vi "GT Get Pos.vi"(8 "error in (no error)":errorcluster caption="错误输入（无错误）", 9 "pPos":i32, 10 "profile":i16, 11 "cardNum":i16) -> (0 "error out":errorcluster caption="错误输出", 1 "pPos out":i32, 3 "function return":i16)   [LabVIEW 2014, in "gts.lvlib"]
doc: "GT_API GT_GetPos(short cardNum,short profile,long *pPos);"
uses:
  gts.lvlib
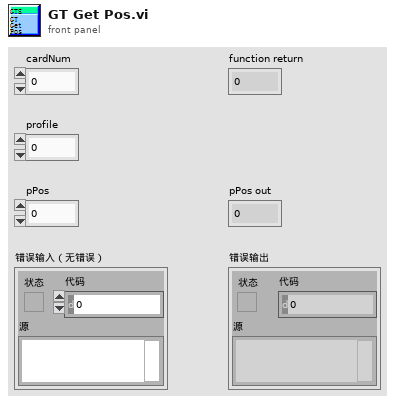
[diagram p1: front panel]
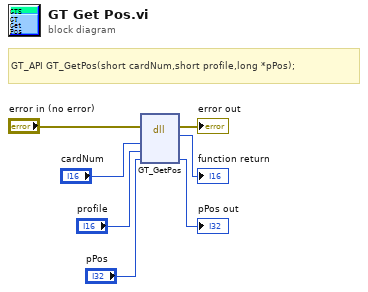
[diagram p0: block diagram]
diagram:
  # "GT_API GT_GetPos(short cardNum,short profile,long *pPos);"
  n1 = dll-call lib="PTH2habs D固高科技资料GTS控制卡GTS卡18年上半年资料dllVC32bit\nmulti_cardgts.*" fn="GT_GetPos"(error in="error in (no error)", "cardNum"="cardNum", "profile"="profile", "pPos"="pPos") -> (error out=→"error out":errorcluster, →"function return":i16, "pPos"=→"pPos out":i32)  [unwired: 4 in, 1 out]
